vi "I16ToString(cast).vi"(1 "I16":i16 format="DEC:%2d\nHEX:%2x") -> (0 "String":string)   [LabVIEW 2012]
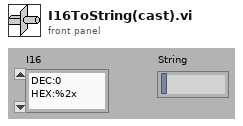
[diagram p1: front panel]
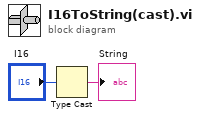
[diagram p0: block diagram]
diagram:
  n1 = Type Cast(x="I16") -> (*(type *) &x=→"String":string)  [unwired: 1 in]
